vi "USB Read User Data.vi"(9 "DataLen":i32, 10 "OffsetAddr":i32, 11 "DevIndex":i32) -> (2 "function return":bool, 3 "pReadData":u8[](array[numeric]))   [LabVIEW 2010, in "usb_device.lvlib"]
doc: "bool WINAPI USB_ReadUserData(int DevIndex,int OffsetAddr,unsigned char *pReadData,int DataLen);"
uses:
  usb_device.lvlib
  USB2XXX.dll
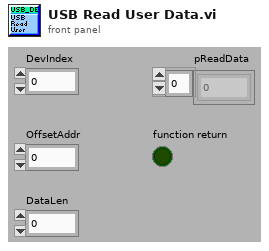
[diagram p1: front panel]
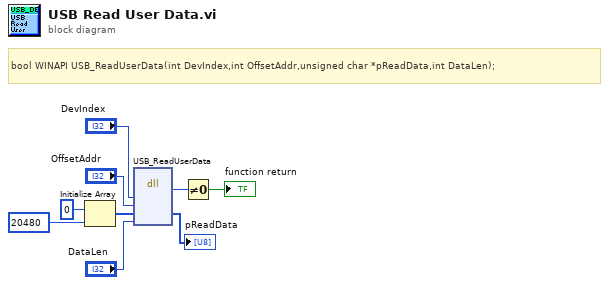
[diagram p0: block diagram]
diagram:
  # "bool WINAPI USB_ReadUserData(int DevIndex,int OffsetAddr,unsigned char *pReadData,int DataLen);"
  n1 = Initialize Array(u8 0 ("element"), 20480 ("dimension size")) -> (w5:u8[])
  n2 = dll-call lib="G:/OtherWork/USB2XXX_Example/trunk/Labview/PublicFiles/usb_device/USB2XXX.*" fn="USB_ReadUserData"("DevIndex"="DevIndex", "OffsetAddr"="OffsetAddr", "pReadData"=w5, "DataLen"="DataLen") -> (w8:u8, "pReadData"=→"pReadData":u8[])  [unwired: 6 in, 2 out]
  n3 = Not Equal To 0?(x=w8) -> (x != 0?=→"function return":bool)
